vi "Gergberg Saxton.vi"() -> ()   [LabVIEW 2012, in "LightPipes.lvlib"]
uses:
  LightPipes.lvlib
panel:
  in  "distance":dbl=1.0
  in  "Number of Iteration":i32
  out "Iteration":i32
  out "field out":T1
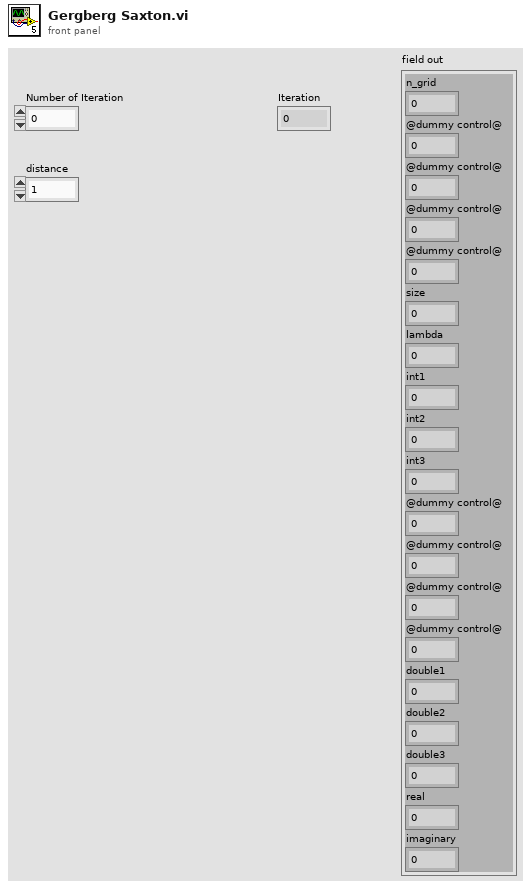
[diagram p1: front panel]
types:
  T1 = cluster{"n_grid":i32, "@dummy control@":i8, "@dummy control@":i8, "@dummy control@":i8, "@dummy control@":i8, "size":dbl, "lambda":dbl, "int1":i32, "int2":i32, "int3":i32, "@dummy control@":i8, "@dummy control@":i8, "@dummy control@":i8, "@dummy control@":i8, "double1":dbl, "double2":dbl, "double3":dbl, "real":u32, "imaginary":u32}
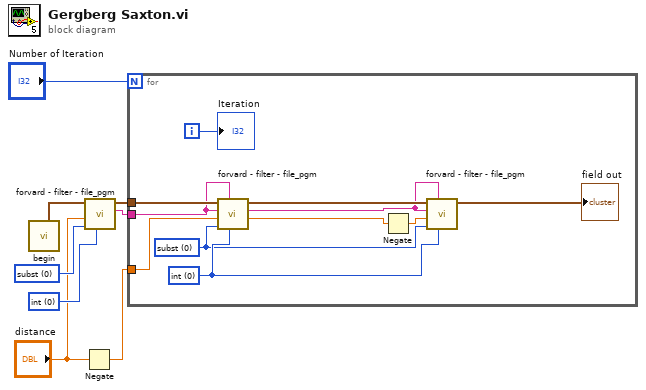
[diagram p0: block diagram]
diagram:
  w5 = i16 0 items=["subst", "mult"] ("c2")
  w6 = i16 0 items=["int", "pha"] ("c1")
  n1 = call "begin.vi"() -> ("field out"=w7:T1)  [unwired: 11 in]
  n2 = Negate(x="distance") -> (-x=w3:dbl)
  n3 = call "forvard - filter - file_pgm.vi"("intensity/phase"=w6, "multiplication/substitution"=w5, "forward distance"="distance", "field"=w7) -> ("path pgm out"=w4:string, "field out"=w1:T1)  [unwired: 4 in, 1 out]
  n4 = for {
    N: "Number of Iteration" -> [_]
    tunnel: w1 -> [w18]
    tunnel: w4 -> [w10]
    tunnel: w3 -> [w11]
    i -> [w19]
    w12 = i16 0 items=["subst", "mult"] ("multiplication/substitution")
    w13 = i16 0 items=["int", "pha"] ("intensity/phase")
    n5 = call "forvard - filter - file_pgm.vi"("intensity/phase"=w13, "path filter in"=w10, "multiplication/substitution"=w12, "forward distance"=w11, "path pgm in"=w10, "field"=w18) -> ("forwarded dist"=w15:dbl, "path pgm out"=w9:string, "field out"=w17:T1)  [unwired: 2 in]
    n6 = Negate(x=w15) -> (-x=w14:dbl)
    n7 = call "forvard - filter - file_pgm.vi"("intensity/phase"=w13, "path filter in"=w9, "multiplication/substitution"=w12, "forward distance"=w14, "path pgm in"=w9, "field"=w17) -> ("field out"=→"field out":T1)  [unwired: 2 in, 2 out]
    "Iteration" <- w19
  }
